vi "GDX_ACC_AccelPitchRoll.vi"(9 "z Accel":dbl, 10 "y Accel":dbl, 11 "x Accel":dbl) -> (2 "Roll":dbl, 3 "Pitch":dbl)   [LabVIEW 2019]
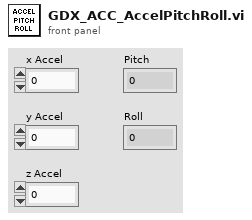
[diagram p1: front panel]
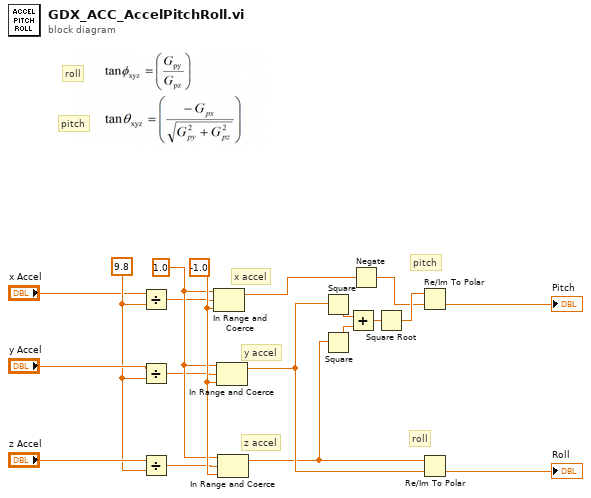
[diagram p0: block diagram]
diagram:
  w17 = 9.8 ("y")
  w7 = -1.0 ("lower limit")
  w6 = 1.0 ("upper limit")
  # "pitch"
  # "roll"
  # "roll"
  # "pitch"
  # "z accel"
  # "y accel"
  # "x accel"
  n1 = Divide(x="x Accel", y=w17) -> (x/y=w3:dbl)
  n2 = Divide(x="y Accel", y=w17) -> (x/y=w4:dbl)
  n3 = Divide(x="z Accel", y=w17) -> (x/y=w5:dbl)
  n4 = In Range and Coerce(upper limit=w6, x=w3, lower limit=w7) -> (coerced(x)=w15:dbl)  [unwired: 1 out]
  n5 = In Range and Coerce(upper limit=w6, x=w4, lower limit=w7) -> (coerced(x)=w14:dbl)  [unwired: 1 out]
  n6 = In Range and Coerce(upper limit=w6, x=w5, lower limit=w7) -> (coerced(x)=w11:dbl)  [unwired: 1 out]
  n7 = Square(x=w14) -> (x^2=w8:dbl)
  n8 = Square(x=w11) -> (x^2=w9:dbl)
  n9 = Add(x=w8, y=w9) -> (x+y=w10:dbl)
  n10 = Negate(x=w15) -> (-x=w12:dbl)
  n11 = Square Root(x=w10) -> (sqrt(x)=w13:dbl)
  n12 = Re/Im To Polar(2:w12, 3:w13) -> (0:→"Pitch":dbl)  [unwired: 1 out]
  n13 = Re/Im To Polar(2:w14, 3:w11) -> (0:→"Roll":dbl)  [unwired: 1 out]
